vi "Read useUTC.vi"(8 "error in (no error)":errorcluster, 11 "Layout in":refnum<class "Layout.lvclass">) -> (0 "error out":errorcluster, 2 "useUTC":bool, 3 "Layout out":refnum<class "Layout.lvclass">)   [LabVIEW 2026, in "Lumberjack.lvlib" / "Layout.lvclass"]
doc: "Returns the layout's useUTC flag.\nClass private-data accessor; reads the `useUTC` field so a concrete Format frames its timestamp in UTC (TRUE) or local time (FALSE). No side effects.\nLumberjack.lvlib, Layout.lvclass, protected."
uses:
  Layout.lvclass
  Layout.lvclass/Layout.ctl
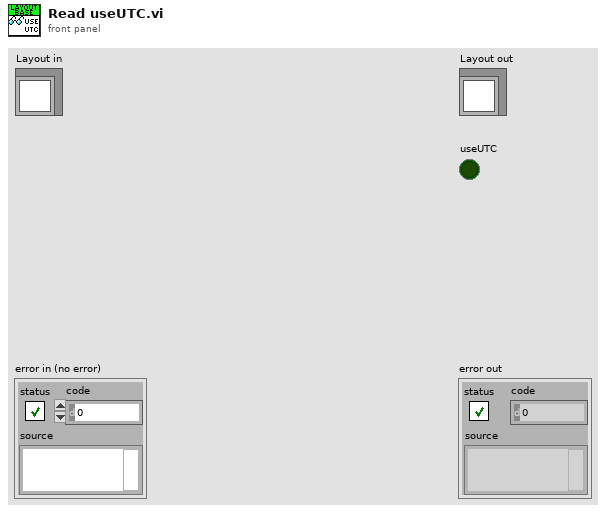
[diagram p1: front panel]
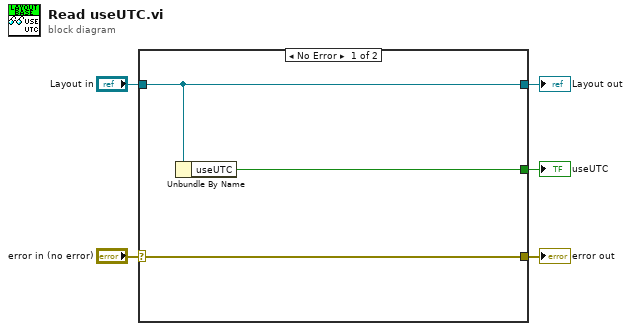
[diagram p0: block diagram]
diagram:
  n1 = case shown="No Error" "error in (no error)" {
    selector: "error in (no error)" -> [w8 w9]
    tunnel: [w8 w9] -> w4
    tunnel: [w7 w10] -> w2
    tunnel: "Layout in" -> [w7 w10]
    tunnel: [w6 _] -> w1
    frame No Error {
      n2 = Unbundle By Name(w7) -> ("useUTC"=w6:bool)
    }
    frame Error {
    }
  }
  "error out" <- w4
  "Layout out" <- w2
  "useUTC" <- w1
